vi "Constructor.vi"(8 "error in (no error)":errorcluster, 11 "Top Level Diagram":refnum<vi>) -> (0 "error out":errorcluster, 3 "Block Diagram":refnum<class "Block Diagram.lvclass">)   [LabVIEW 2015, in "Block Diagram.lvclass"]
uses:
  Block Diagram.lvclass
  Main Sequence/Main Sequence.lvclass
  DMA Loop/DMA Loop.lvclass
  Block Diagram.lvclass/Block Diagram.ctl
  Module Loop/Module Loop.lvclass
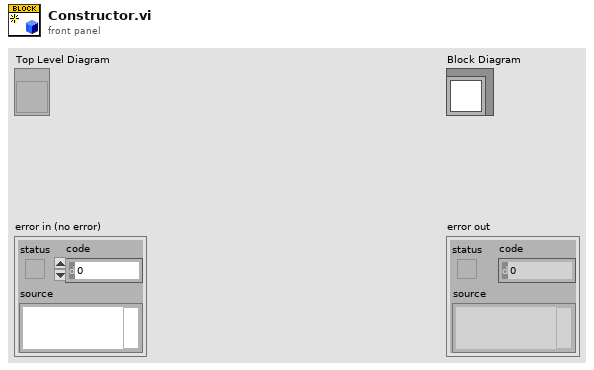
[diagram p1: front panel]
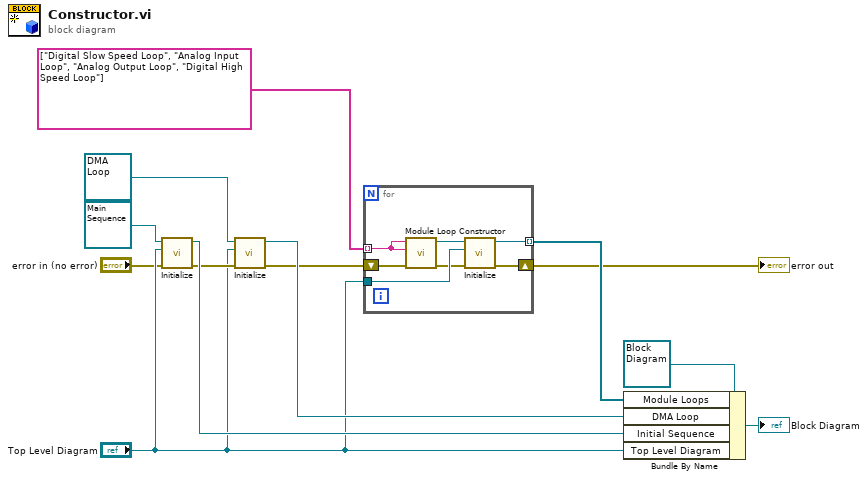
[diagram p0: block diagram]
diagram:
  n1 = call-dynamic "Initialize.vi"("error in (no error)"="error in (no error)", "Top Level Diagram"="Top Level Diagram", "Initial Sequence in"=refnum<class "Main Sequence.lvclass"> refnum ("Initial Sequence.lvclass")) -> ("error out"=w8:errorcluster, "Initial Sequence out"=w9:refnum<class "Main Sequence.lvclass">)  [unwired: 7 in]
  n2 = call-dynamic "Initialize.vi"("error in (no error)"=w8, "Top Level Diagram"="Top Level Diagram", "DMA Loop in"=refnum<class "DMA Loop.lvclass"> refnum ("DMA Loop.lvclass")) -> ("error out"=w3:errorcluster, "DMA Loop out"=w10:refnum<class "DMA Loop.lvclass">)  [unwired: 7 in]
  n3 = for {
    tunnel: "Top Level Diagram" -> [w19]
    shift-right: [w20] -> w2
    shift-left: w3 -> [w16]
    tunnel: [w18] -> w4 mode=indexing
    tunnel: string[] ["Digital Slow Speed Loop", "Analog Input Loop", "Analog Output Loop", "Digital High Speed Loop"] -> [w14] mode=indexing
    n4 = call "Module Loop Constructor.vi"("error in (no error)"=w16, "Name"=w14, "Type"=w14) -> ("error out"=w15:errorcluster, "Module Loop.lvclass"=w17:refnum<class "Module Loop.lvclass">)  [unwired: 7 in]
    n5 = call-dynamic "Initialize.vi"("error in (no error)"=w15, "Top Level Diagram"=w19, "IO Loop in"=w17) -> ("error out"=w20:errorcluster, "IO Loop out"=w18:refnum<class "Module Loop.lvclass">)  [unwired: 7 in]
  }
  "error out" <- w2
  n6 = Bundle By Name(cluster=refnum<class "Block Diagram.lvclass"> refnum ("Block Diagram.lvclass"), "Module Loops"=w4, "DMA Loop"=w10, "Initial Sequence"=w9, "Top Level Diagram"="Top Level Diagram") -> (→"Block Diagram":refnum<class "Block Diagram.lvclass">)
